vi "Get cif_channelcore_Direction.vi"(8 "error in (no error)":errorcluster, 11 "gRPCid":T1) -> (0 "error out":errorcluster, 2 "package_template_enum":T2, 3 "gRPCid out":T1)   [LabVIEW 2021, in "CIFCoreChannel_server.lvlib"]
uses:
  CIFCoreChannel_server.lvlib
  cif_channelcore_Direction.ctl
  <vilib>/gRPC/LabVIEW gRPC Library/Shared/grpcId.ctl
  2ed25e12-861d-4677-8ead-ace2906b2041.vi
  <vilib>/gRPC/LabVIEW gRPC Library/Shared/TranslateGrpcError.vi
  <vilib>/gRPC/LabVIEW gRPC Library/Server API/Server/Get Server DLL Path.vi
  <vilib>/Utility/error.llb/Error Cluster From Error Code.vi
  <vilib>/gRPC/LabVIEW gRPC Library/grpc-lvsupport-release.lvlib
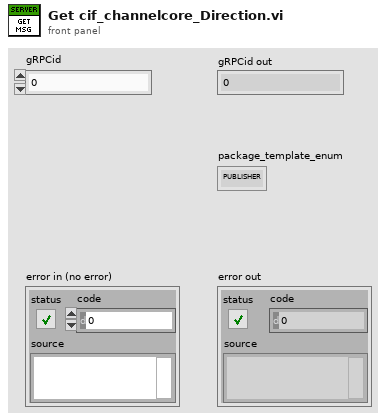
[diagram p1: front panel]
types:
  T1 = typedef "grpc-lvsupport-release.lvlib/grpcId.ctl" = u64
  T2 = typedef "CIFCoreChannel_server.lvlib/cif_channelcore_Direction.ctl" = enum32{"PUBLISHER", "SUBSCRIBER"}
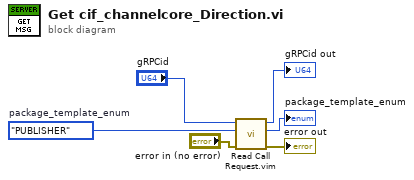
[diagram p0: block diagram]
diagram:
  w2 = cif_channelcore_Direction."PUBLISHER"  # package_template_enum
  n1 = call "Read Call Request.vim"("error in"="error in (no error)", "Request Type"=w2, "gRPCid in"="gRPCid") -> ("error out"=→"error out":errorcluster, "Request Data"=→"package_template_enum":T2, "gRPCid out"=→"gRPCid out":T1)  [unwired: 6 in]
